vi "SECoP_dataModifyBool.vi"(6 "Value":bool, 7 "Position":u32, 8 "error in (no error)":errorcluster, 9 "Index":u32, 10 "SECoP_dataPtr":T1 {"ptr64" format="%.0x"; "ptr32" format="%.0x"}, 11 "DLL path (in)":T2) -> (0 "error out":errorcluster, 3 "DLL path (out)":T2)   [LabVIEW 2023, in "SECoP.lvlib"]
doc: "Call <b>\"SECoP_dataModifyBool.vi\"</b> to change the value of a boolean (SECoP_dataPtr).\n\n<b>DLL path</b> input and output of cluster from \"SECoP-Initialize.vi\"\n<b>SECoP_dataPtr</b> data to access\n<b>Position</b> points to a virtual flattened entry of the data type\n<b>Index</b> zero based index into array type or 0 for single type\n<b>Value</b> new boolean value"
uses:
  SECoP.lvlib
  SECoP-libraries.ctl
  SECoP-data.ctl
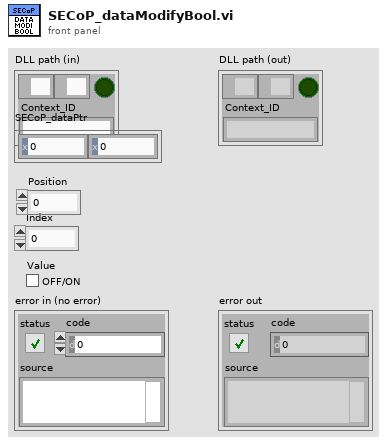
[diagram p1: front panel]
types:
  T1 = typedef "SECoP.lvlib/SECoP-data.ctl" = cluster{"ptr32":u32, "ptr64":u64}
  T2 = typedef "SECoP.lvlib/SECoP-libraries.ctl" = cluster{"serverDLL":path, "variantDLL":path, "cleanup_mode":bool, "Context_ID":string}
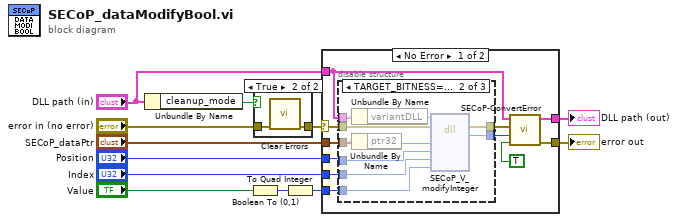
[diagram p0: block diagram]
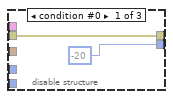
[diagram p2: hidden frame]
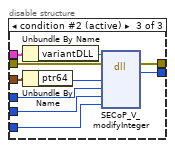
[diagram p3: hidden frame]
diagram:
  n1 = Unbundle By Name("DLL path (in)") -> ("cleanup_mode"=w9:bool)
  n2 = Boolean To (0,1)(Boolean="Value") -> (0, 1=w2:i16)
  n3 = case shown="True" w9 {
    tunnel: "error in (no error)" -> [w13 w15]
    tunnel: [w13 w14] -> w7
    frame False {
    }
    frame True {
      n4 = call <vilib>:"Clear Errors.vi"("error in (no error)"=w15) -> ("error out"=w14:errorcluster)  [unwired: 5 in, 1 out]
    }
  }
  n5 = To Quad Integer(1:w2) -> (0:w1:i64)
  n6 = case shown="No Error" w7 {
    selector: w7 -> [w22 w49]
    tunnel: "DLL path (in)" -> [w16 w50]
    tunnel: [w25 w50] -> w11
    tunnel: [w26 w49] -> w10
    tunnel: "Index" -> [w19 _]
    tunnel: w1 -> [w20 _]
    tunnel: "Position" -> [w18 _]
    tunnel: "SECoP_dataPtr" -> [w21 _]
    frame No Error {
      n7 = disable-structure shown="TARGET_BITNESS==32" {
        disable-tunnel: [w28 w38 w48] -> w23
        disable-tunnel: w16 -> [_ w37 w47]
        disable-tunnel: w22 -> [w28 w36 w46]
        disable-tunnel: w21 -> [_ w35 w45]
        disable-tunnel: w20 -> [_ w33 w43]
        disable-tunnel: w19 -> [_ w32 w42]
        disable-tunnel: w18 -> [_ w31 w41]
        disable-tunnel: [-20 w30 w40] -> w17
        frame condition #0 {
        }
        frame condition #1 {
          n8 = Unbundle By Name(w37) -> ("variantDLL"=w29:path)
          n9 = Unbundle By Name(w35) -> ("ptr32"=w34:u32)
          n10 = dll-call lib="Z:/Praktische_Aufgaben/SECoP-LabVIEW2015/32bit/SECoP32.dll" fn="SECoP_V_modifyInteger"(path in=w29, error in=w36, "Data"=w34, "Position"=w31, "Index"=w32, "Value"=w33) -> (error out=w38:errorcluster, "return type"=w30:i32)  [unwired: 5 in, 1 out]
        }
        frame condition #2 (active) {
          n11 = Unbundle By Name(w47) -> ("variantDLL"=w39:path)
          n12 = Unbundle By Name(w45) -> ("ptr64"=w44:u64)
          n13 = dll-call lib="Z:/Praktische_Aufgaben/SECoP-LabVIEW2015/32bit/SECoP32.dll" fn="SECoP_V_modifyInteger"(path in=w39, error in=w46, "Data"=w44, "Position"=w41, "Index"=w42, "Value"=w43) -> (error out=w48:errorcluster, "return type"=w40:i32)  [unwired: 5 in, 1 out]
        }
      }
      n14 = call "SECoP-ConvertError.vi"("return is boolean"=TRUE, "return code"=w17, "error in (no error)"=w23, "DLL path (in)"=w16) -> ("error out"=w26:errorcluster, "DLL path (out)"=w25:T2)  [unwired: 6 in]
    }
    frame Error {
    }
  }
  "DLL path (out)" <- w11
  "error out" <- w10
